vi "subAddProjectItems.vi"(8 "error in (no error)":errorcluster, 9 "ProjectItems":refnum<class "ProjectItem.lvclass">[](array[class]), 10 "Owning project":path, 11 "SolutionBuilder in":refnum<class "SolutionBuilder.lvclass">) -> (0 "error out":errorcluster, 3 "SolutionBuilder out":refnum<class "SolutionBuilder.lvclass">)   [LabVIEW 2020, in "SolutionBuilder.lvlib" / "SolutionBuilder.lvclass"]
uses:
  SolutionBuilder.lvclass
  ProjectItem/ProjectItem.lvclass
  SolutionBuilder.lvclass/SolutionBuilder.ctl
  <vilib>/Utility/miscctls.llb/LVMapReplaceAction.ctl
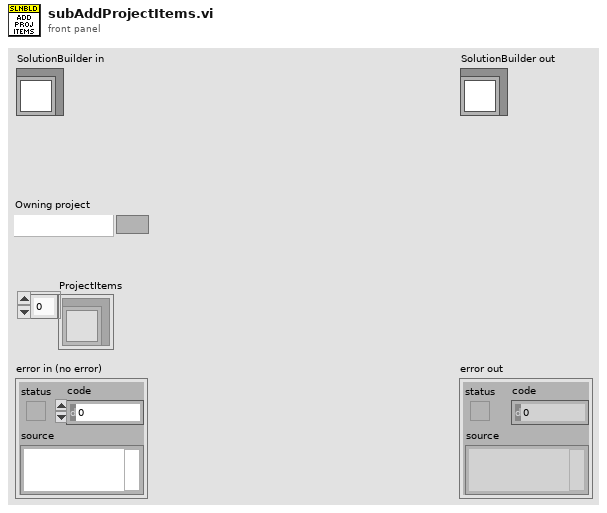
[diagram p1: front panel]
types:
  T1 = typedef "LVMapReplaceAction.ctl" = enum32{"Modify Entry only if found", "Add or Modify Entry", "Delete Entry"}
  T2 = typedef "SolutionBuilder.lvlib/SolutionBuilder.lvclass/ProjectItemMap.ctl" = map{path, refnum<class "ProjectItem.lvclass">[]}
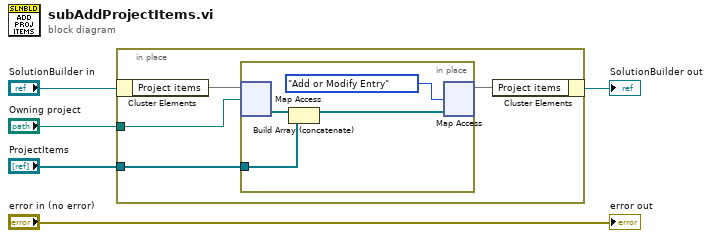
[diagram p0: block diagram]
diagram:
  n1 = in-place {
    in-place-border: "Owning project" -> [w7]
    in-place-border: "ProjectItems" -> [w9]
    n2 = in-place-cluster #1("SolutionBuilder in") -> ("Project items"=w8:T2)
    n3 = in-place {
      in-place-border: w9 -> [w12]
      n4 = in-place-map #2(w8, w7) -> (w13:refnum<class "ProjectItem.lvclass">[])  [unwired: 1 in, 1 out]
      n5 = Build Array (concatenate)(w13, w12) -> (w11:refnum<class "ProjectItem.lvclass">[])
      n6 = in-place-map #2(w11, LVMapReplaceAction."Add or Modify Entry" ("action")) -> (w6:T2)  [unwired: 2 out]
    }
    n7 = in-place-cluster #1("Project items"=w6) -> (→"SolutionBuilder out":refnum<class "SolutionBuilder.lvclass">)
  }
  "error out" <- "error in (no error)"
